vi "Read Multi Eval Meas ES Flatness Results.vi"(8 "error in (no error)":errorcluster, 9 "Result Type (Current)":i32(ring) items=["Current", "Average", "Extreme", "Standard Deviation"], 10 "Instance (1)":T2=1, 11 "VISA resource name":refnum<visa-resource-name>) -> (0 "error out":errorcluster, 1 "ES Flatness Results":T1 {"Max R2" format="%^.3e"; "Min R2" format="%^.3e"; "Max R1" format="%^.3e"; "Min R1" format="%^.3e"; "Max R2 Min R1" format="%^.3e"; "Max R1 Min R2" format="%^.3e"; "Ripple 2" format="%^.3e"; "Ripple 1" format="%^.3e"; "Out Of Tolerance" format="%^.3e"}, 2 "Reliability":i32, 3 "VISA resource name out":refnum<visa-resource-name>)   [LabVIEW 2020, in "Rohde&Schwarz CMXP NR FR2 Measurement.lvlib"]
doc: "Starts a new single shot measurement and returns the multi eval measurement ES Flatness results.\n\nAttributes:\nRSCMXPNRFR2M_ATTR_READ_MULTI_EVAL_MEASUREMENT_ESF_AVERAGE_RESULTS\nRSCMXPNRFR2M_ATTR_READ_MULTI_EVAL_MEASUREMENT_ESF_CURRENT_RESULTS\nRSCMXPNRFR2M_ATTR_READ_MULTI_EVAL_MEASUREMENT_ESF_EXTREME_RESULTS\nRSCMXPNRFR2M_ATTR_READ_MULTI_EVAL_MEASUREMENT_ESF_STANDARD_DEVIATION_RESULTS\n\nRemote-control commands:\nREAD:NRMMw:MEAS<i>:MEValuation:ESFLatness:AVERage?\nREAD:NRMMw:MEAS<i>:MEValuation:ESFLatness:CURRent?\nREAD:NRMMw:MEAS<i>:MEValuation:ESFLatness:EXTReme?\nREAD:NRMMw:MEAS<i>:MEValuation:ESFLatness:SDEViation?"
uses:
  <instrlib>/Rohde&Schwarz CMXP NR FR2 Measurement/Rohde&Schwarz CMXP NR FR2 Measurement.lvlib
  <instrlib>/Rohde&Schwarz CMXP NR FR2 Measurement/Private/_Instance.ctl
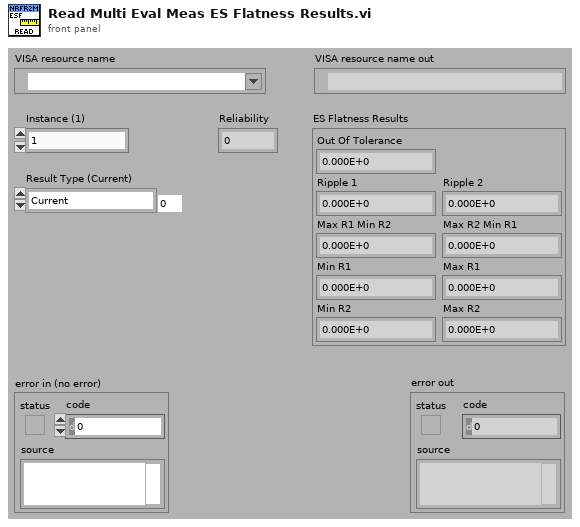
[diagram p1: front panel]
types:
  T1 = cluster{"Out Of Tolerance":dbl, "Ripple 1":dbl, "Ripple 2":dbl, "Max R1 Min R2":dbl, "Max R2 Min R1":dbl, "Min R1":dbl, "Max R1":dbl, "Min R2":dbl, "Max R2":dbl}
  T2 = typedef "Rohde&Schwarz CMXP NR FR2 Measurement.lvlib/_Instance.ctl" = i32
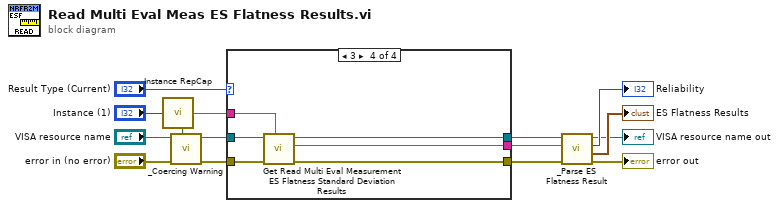
[diagram p0: block diagram]
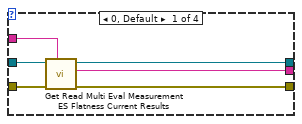
[diagram p2: hidden frame]
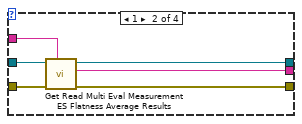
[diagram p3: hidden frame]
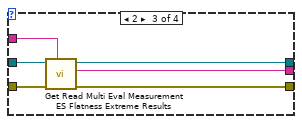
[diagram p4: hidden frame]
diagram:
  n1 = call <instrlib>:"Instance RepCap.vi"("Instance In"="Instance (1)") -> ("In Range?"=w2:bool, "RepCap Identifier Out"=w14:string)  [unwired: 1 in]
  n2 = call <instrlib>:"_Coercing Warning.vi"("In Range?"=w2, "error in (no error)"="error in (no error)", "VISA resource name"="VISA resource name") -> ("error out"=w3:errorcluster, "VISA resource name out"=w4:refnum<visa-resource-name>)  [unwired: 7 in]
  n3 = case shown="3" "Result Type (Current)" {
    tunnel: w3 -> [w21 w27 w31 w39]
    tunnel: w4 -> [w20 w26 w30 w38]
    tunnel: [w19 w25 w29 w37] -> w10
    tunnel: [w18 w24 w28 w36] -> w9
    tunnel: w14 -> [w17 w23 w33 w35]
    tunnel: [w16 w22 w32 w34] -> w13
    frame 0, Default {
      n4 = call "Get Read Multi Eval Measurement ES Flatness Current Results"("Repeated Capabilities"=w17, "error in (no error)"=w21, "instrument handle"=w20) -> ("error out"=w19:errorcluster, "Read Multi Eval Measurement ES Flatness Current Results"=w16:string, "instrument handle out"=w18:refnum<visa-resource-name>)  [unwired: 6 in]
    }
    frame 1 {
      n5 = call "Get Read Multi Eval Measurement ES Flatness Average Results"("Repeated Capabilities"=w23, "error in (no error)"=w27, "instrument handle"=w26) -> ("error out"=w25:errorcluster, "Read Multi Eval Measurement ES Flatness Average Results"=w22:string, "instrument handle out"=w24:refnum<visa-resource-name>)  [unwired: 6 in]
    }
    frame 2 {
      n6 = call "Get Read Multi Eval Measurement ES Flatness Extreme Results"("Repeated Capabilities"=w33, "error in (no error)"=w31, "instrument handle"=w30) -> ("error out"=w29:errorcluster, "Read Multi Eval Measurement ES Flatness Extreme Results"=w32:string, "instrument handle out"=w28:refnum<visa-resource-name>)  [unwired: 6 in]
    }
    frame 3 {
      n7 = call "Get Read Multi Eval Measurement ES Flatness Standard Deviation Results"("Repeated Capabilities"=w35, "error in (no error)"=w39, "instrument handle"=w38) -> ("error out"=w37:errorcluster, "Read Multi Eval Measurement ES Flatness Standard Deviation Results"=w34:string, "instrument handle out"=w36:refnum<visa-resource-name>)  [unwired: 6 in]
    }
  }
  n8 = call <instrlib>:"_Parse ES Flatness Result.vi"("error in (no error)"=w10, "Input String"=w13, "VISA resource name"=w9) -> ("error out"=→"error out":errorcluster, "Results"=→"ES Flatness Results":T1, "Reliability"=→"Reliability":i32, "VISA resource name out"=→"VISA resource name out":refnum<visa-resource-name>)  [unwired: 5 in]
